vi "Tamaño de BD.vi"() -> ()   [LabVIEW 2018]
uses:
  <vilib>/RAFA Solutions/Harmony UI Controls Kit/Numeric/Numeric Indicator.ctl
  <vilib>/RAFA Solutions/Harmony UI Controls Kit/Boolean/Blank Button - Red.ctl
  <vilib>/addons/database/Connection.llb/DB Tools Open Connec (Path).vi
  <vilib>/addons/database/Connection.llb/Conn Execute.vi
  <vilib>/addons/database/Recordset.llb/Rec Fetch Recordset Data (R).vi
  <vilib>/addons/database/Recordset.llb/Rec Destroy - Connection.vi
  <vilib>/addons/database/_DB Variant To Data/Database Variant To Data.xnode
  <vilib>/addons/database/NI_Database_API.lvlib
  <vilib>/RAFA Solutions/Harmony UI Controls Kit/Flat UI Design.lvlib
panel:
  in  "SALIR":T1
  in  "error in":errorcluster
  out "error out":errorcluster
  out "Numeric Indicator":T2
  # "TAMAÑO DE LA BASE DE DATOS"
  # "MB"
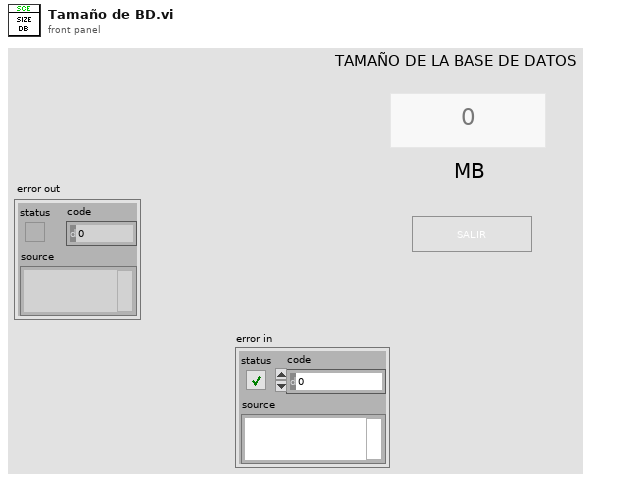
[diagram p1: front panel]
types:
  T1 = typedef "Flat UI Design.lvlib/Blank Button - Red.ctl" = bool
  T2 = typedef "Flat UI Design.lvlib/Numeric Indicator.ctl" = sgl
  T3 = typedef "NI_Database_API.lvlib/Conn ObjectReference.ctl" = refnum<k1>
  T4 = typedef "NI_Database_API.lvlib/Rec ObjectReference.ctl" = refnum<k1>
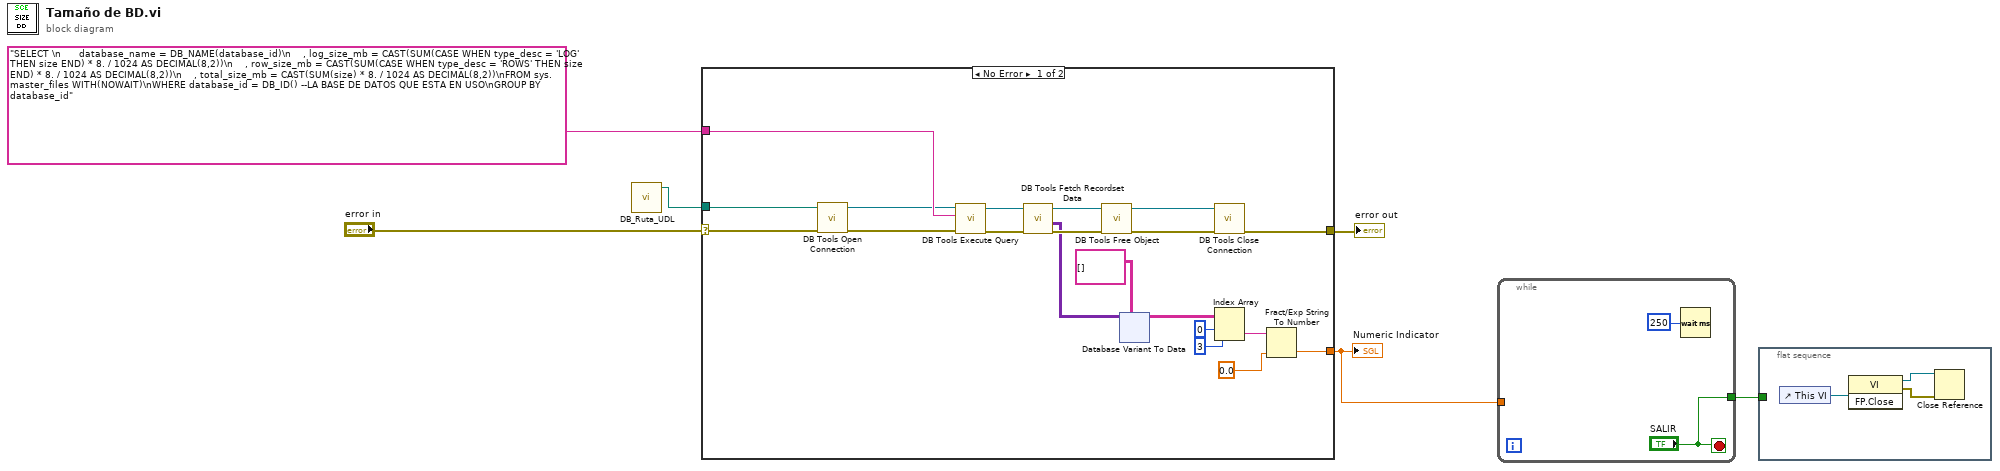
[diagram p0: block diagram]
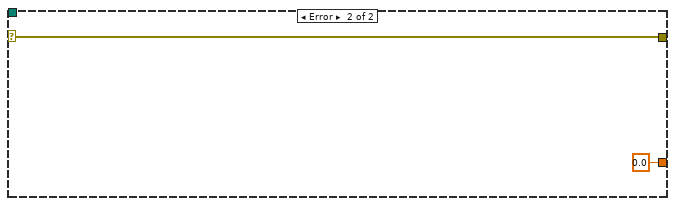
[diagram p2: hidden frame]
diagram:
  n1 = call "DB_Ruta_UDL.vi"() -> ("UDL ruta"=w1:path)  [unwired: 11 in]
  n2 = case shown="No Error" "error in" {
    selector: "error in" -> [w24 w72]
    tunnel: [w18 w72] -> w6
    tunnel: "SELECT \n      database_name = DB_NAME(database_id)\n    , log_size_mb = CAST(SUM(CASE WHEN type_desc = 'LOG' THEN size END) * 8. / 1024 AS DECIMAL(8,2))\n    , row_size_mb = CAST(SUM(CASE WHEN type_desc = 'ROWS' THEN size END) * 8. / 1024 AS DECIMAL(8,2))\n    , total_size_mb = CAST(SUM(size) * 8. / 1024 AS DECIMAL(8,2))\nFROM sys.master_files WITH(NOWAIT)\nWHERE database_id = DB_ID() --LA BASE DE DATOS QUE ESTA EN USO\nGROUP BY database_id" ("SQL") -> [w23 _]
    tunnel: [w10 sgl 0.0] -> w3
    tunnel: w1 -> [w8 _]
    frame No Error {
      n3 = call-poly <vilib>:"DB Tools Open Connection.vi"("error in (no error)"=w24, "connection information"=w8) -> ("error out"=w19:errorcluster, "connection reference"=w15:T3)  [unwired: 6 in]
      n4 = call-poly <vilib>:"DB Tools Execute Query.vi"("error in (no error)"=w19, "SQL query"=w23, "connection reference"=w15) -> ("error out"=w25:errorcluster, "recordset reference"=w22:T4)  [unwired: 5 in]
      n5 = call-poly <vilib>:"DB Tools Fetch Recordset Data.vi"("error in (no error)"=w25, "recordset reference"=w22) -> ("error out"=w20:errorcluster, "recordset data"=w17:variant[][], "recordset reference out"=w21:T4)  [unwired: 3 in]
      n6 = call-poly <vilib>:"DB Tools Free Object.vi"("error in (no error)"=w20, "recordset reference"=w21) -> ("error out"=w26:errorcluster, "connection reference"=w7:T3)  [unwired: 8 in]
      n7 = xnode "Database Variant To Data"("database variant"=w17, "type"=string[][] []) -> ("data"=w14:string[][])  [unwired: 1 in, 1 out]
      n8 = call <vilib>:"DB Tools Close Connection.vi"("error in (no error)"=w26, "connection reference"=w7) -> ("error out"=w18:errorcluster)  [unwired: 5 in]
      n9 = Index Array(array=w14, index (row)=0, index (col)=3 ("disabled index (col)")) -> (element=w11:string)
      n10 = Fract/Exp String To Number(string=w11, default (0 dbl)=T2 0.0 ("Numeric Indicator")) -> (number=w10:sgl)  [unwired: 2 in, 1 out]
    }
    frame Error {
    }
  }
  "Numeric Indicator" <- w3
  "error out" <- w6
  n11 = while {
    tunnel: w3 -> [_]
    tunnel: ["SALIR"] -> w2
    stop <- "SALIR" stop-if-true
    n12 = Wait (ms)(milliseconds to wait=u32 250 ("Wait time (msec)")) -> ()  [unwired: 1 out]
  }
  n13 = flat-sequence {
    tunnel: w2 -> [_]
    frame #0 {
      n14 = control-ref of="This VI"() -> (w77:refnum<vi>)
      n15 = invoke class="VI" method="FP.Close"(reference=w77) -> (reference out=w76:refnum<vi>, error out=w75:errorcluster)  [unwired: 2 in, 1 out]
      n16 = Close Reference(reference=w76, error in (no error)=w75) -> ()  [unwired: 1 out]
    }
  }
